vi "Matrix Operations.vi"() -> ()   [LabVIEW 2011]
uses:
  <vilib>/Analysis/Matrix/Datatypes/RealMatrix.ctl
  <vilib>/Analysis/baseanly.llb/Real Inverse Matrix.vi
  <vilib>/Analysis/7linalg.llb/Real Eigenvalues and Vectors.vi
  <vilib>/Analysis/_algsub.llb/Real Matrix Rank.vi
  <vilib>/Analysis/NI_AALBase.lvlib
  <vilib>/Analysis/NI_AALPro.lvlib
  <vilib>/Analysis/Matrix/NI_Matrix.lvlib
panel:
  in  "Index Column":dbl
  out "Diagonal Matrix":T1
  in  "Index Row":dbl
  in  "Input Matrix":T1
  out "Rank":dbl
  in  "Real Matrix":T1
  out "Array 2":dbl[](array[numeric])
  in  "Array":dbl[][](array[numeric])
  out "INVERSE MATRIX":dbl[][](array[numeric])
  in  "INPUT MATRIX":dbl[][](array[numeric])
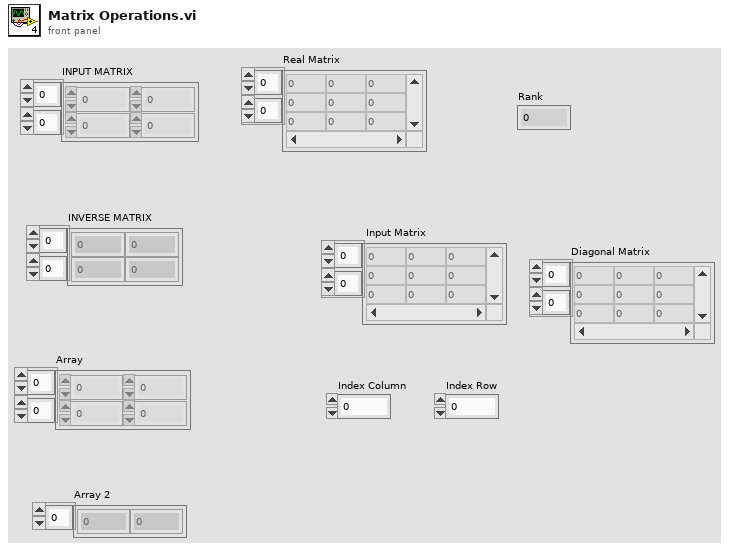
[diagram p1: front panel]
types:
  T1 = typedef "NI_Matrix.lvlib/RealMatrix.ctl" = dbl[][]
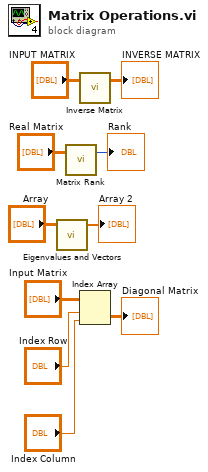
[diagram p0: block diagram]
diagram:
  n1 = call-poly <vilib>:"Eigenvalues and Vectors.vi"("Input Matrix"="Array") -> ("Eigenvalues"=→"Array 2":cdb[])  [unwired: 2 in, 2 out]
  n2 = call-poly <vilib>:"Matrix Rank.vi"("Input Matrix"="Real Matrix") -> ("rank"=→"Rank":i32)  [unwired: 1 in, 1 out]
  n3 = call-poly <vilib>:"Inverse Matrix.vi"("Input Matrix"="INPUT MATRIX") -> ("Inverse Matrix"=→"INVERSE MATRIX":T1)  [unwired: 1 in, 1 out]
  n4 = Index Array(array="Input Matrix", index (row)="Index Row", index (col)="Index Column") -> (element=→"Diagonal Matrix":T1)
